vi "Read Modules Stop Notifier.vi"(8 "error in (no error)":errorcluster, 11 "Root Actor in":refnum<class "Root Actor.lvclass">) -> (0 "error out":errorcluster, 2 "Leaf  Notifier":map{i64[], refnum<class "Notifier.lvclass">}(c390), 3 "Root Actor out":refnum<class "Root Actor.lvclass">)   [LabVIEW 2024, in "Root Actor.lvclass"]
uses:
  Root Actor.lvclass
  Notifier/Notifier.lvclass
  Root Actor.lvclass/Root Actor.ctl
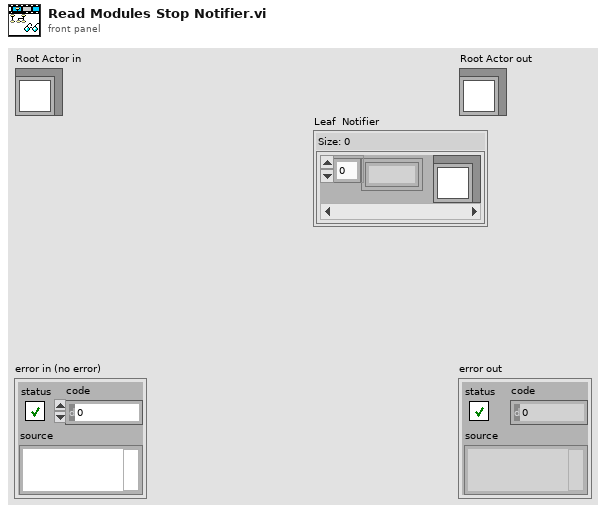
[diagram p1: front panel]
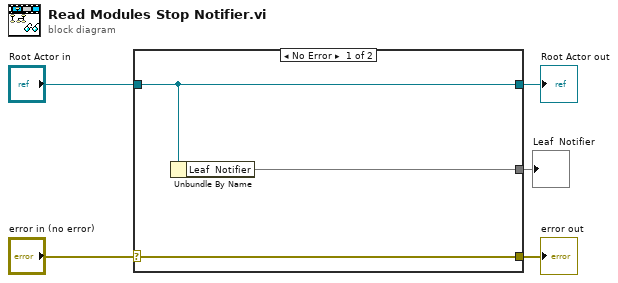
[diagram p0: block diagram]
diagram:
  n1 = case shown="No Error" "error in (no error)" {
    selector: "error in (no error)" -> [w8 w9]
    tunnel: [w8 w9] -> w4
    tunnel: [w7 w10] -> w2
    tunnel: "Root Actor in" -> [w7 w10]
    tunnel: [w6 _] -> w1
    frame No Error {
      n2 = Unbundle By Name(w7) -> ("Leaf  Notifier"=w6:map{i64[], refnum<class "Notifier.lvclass">})
    }
    frame Error {
    }
  }
  "error out" <- w4
  "Root Actor out" <- w2
  "Leaf  Notifier" <- w1
